vi "Load Config.vi"(8 "error in (no error)":errorcluster, 11 "Server Creator Data in":T1) -> (0 "error out":errorcluster, 3 "Server Creator Data out":T1)   [LabVIEW 2025, in "Tools.lvlib"]
uses:
  Tools.lvlib
  Server Creator Data.ctl
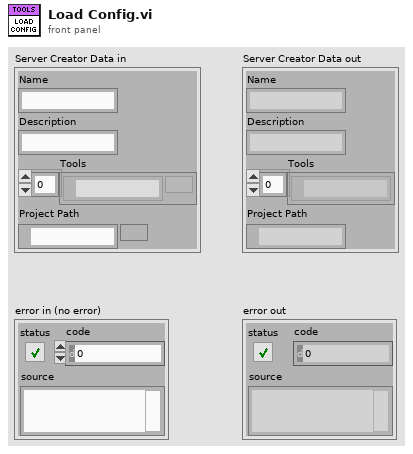
[diagram p1: front panel]
types:
  T1 = typedef "Tools.lvlib/Server Creator Data.ctl" = cluster{"Name":string, "Description":string, "Tools":path[], "Project Path":path}
  T2 = enum16{"open", "replace", "create", "open or create", "replace or create", "replace or create with confirmation"}
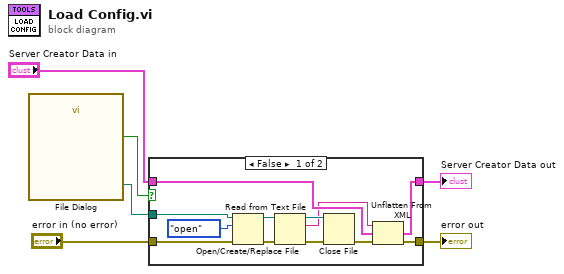
[diagram p0: block diagram]
diagram:
  n1 = call "File Dialog"() -> ("selected path"=w2:path, "cancelled"=w1:bool)  [unwired: 12 in, 2 out]
  n2 = case shown="False" w1 {
    tunnel: "error in (no error)" -> [w14 w19]
    tunnel: "Server Creator Data in" -> [w13 w20]
    tunnel: [w11 w20] -> w4
    tunnel: [w9 w19] -> w3
    tunnel: w2 -> [w8 _]
    frame False {
      n3 = Open/Create/Replace File(file path (use dialog)=w8, error in=w14, operation (0:open)=T2."open") -> (refnum out=w17:refnum<file>, error out=w15:errorcluster)  [unwired: 3 in, 1 out]
      n4 = Read from Text File(file (use dialog)=w17, error in=w15) -> (refnum out=w18:refnum<file>, text=w12:string, error out=w16:errorcluster)  [unwired: 2 in, 1 out]
      n5 = Close File(refnum=w18, error in=w16) -> (error out=w10:errorcluster)  [unwired: 1 out]
      n6 = Unflatten From XML(xml string=w12, type=w13, error in (no error)=w10) -> (value=w11:T1, error out=w9:errorcluster)
    }
    frame True {
    }
  }
  "Server Creator Data out" <- w4
  "error out" <- w3
